vi "Disable Up Down Button.vi"(5 "Length":i32, 7 "Index":i32, 8 "error in (no error)":errorcluster, 9 "Delete Ref":refnum<vi>, 10 "Move Down Ref":refnum<vi>, 11 "Move Up Ref":refnum<vi>) -> (0 "error out":errorcluster)   [LabVIEW 2020, in "3D Plot.lvclass"]
uses:
  3D Plot.lvclass
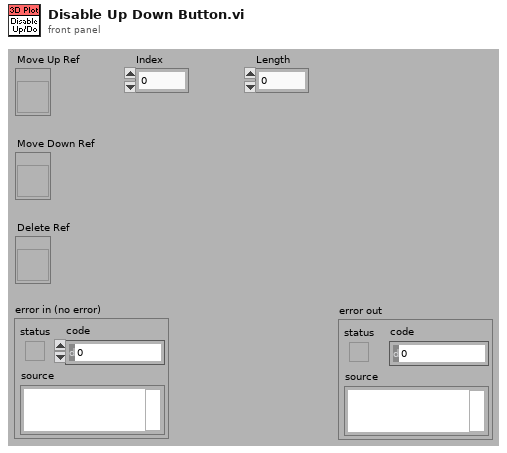
[diagram p1: front panel]
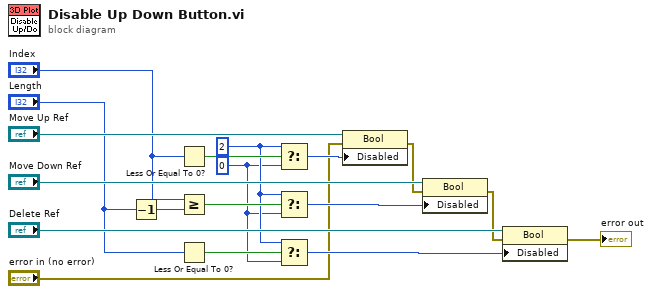
[diagram p0: block diagram]
diagram:
  w8 = u8 2 ("Disabled")
  w7 = u8 0 ("Disabled")
  n1 = Decrement(x="Length") -> (x-1=w10:i32)
  n2 = Less Or Equal To 0?(x="Index") -> (x <= 0?=w16:bool)
  n3 = Greater Or Equal?(x="Index", y=w10) -> (x >= y?=w13:bool)
  n4 = Less Or Equal To 0?(x="Length") -> (x <= 0?=w9:bool)
  n5 = Select(t=w8, s=w16, f=w7) -> (s? t:f=w15:u8)
  n6 = Select(t=w8, s=w13, f=w7) -> (s? t:f=w14:u8)
  n7 = Select(t=w8, s=w9, f=w7) -> (s? t:f=w6:u8)
  n8 = property on="Property Node" class="Bool"(reference="Move Up Ref", error in="error in (no error)", "Disabled"=w15) -> (error out=w12:errorcluster)  [unwired: 1 out]
  n9 = property on="Property Node" class="Bool"(reference="Move Down Ref", error in=w12, "Disabled"=w14) -> (error out=w5:errorcluster)  [unwired: 1 out]
  n10 = property on="Property Node" class="Bool"(reference="Delete Ref", error in=w5, "Disabled"=w6) -> (error out=→"error out":errorcluster)  [unwired: 1 out]
